vi "HDR_Query.vi"(0 "System no.":i32=1 min=1 max=4 step=1, 2 "Section header":string, 5 "error in":errorcluster) -> (14 "Data recorder help string":string, 15 "Lines":string[](array[string]), 16 "Enum values":cluster{"token string":string, i32}[](array[cluster]), 19 "error out":errorcluster)   [LabVIEW 2020]
doc: "Returns help on data recording: possible parameter values for record sources and record trigger options (DRC,DRT), parameters to set and other information. If Section header contains a valid section name, Lines and Enum values return the corresponding section content.\n\nC-887, F-206, M-8X0: Only for GCS syntax version = GCS 2.0 or higher (check with CSV?.vi. If CSV?.vi is not supported, syntax version is GCS 1.0)."
panel:
  # "Get  help for data recorder."
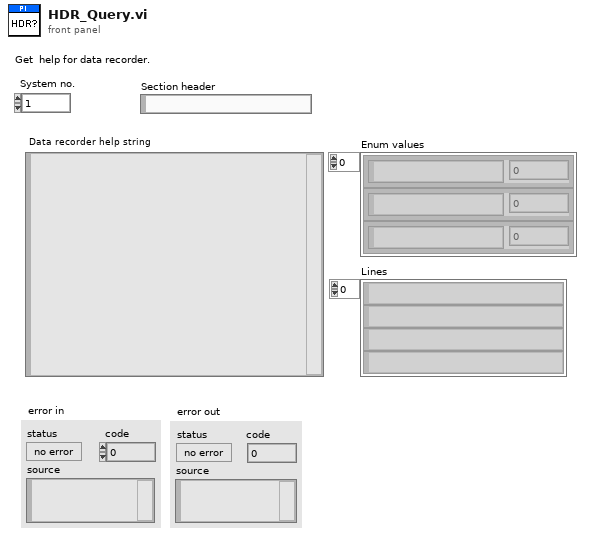
[diagram p1: front panel]
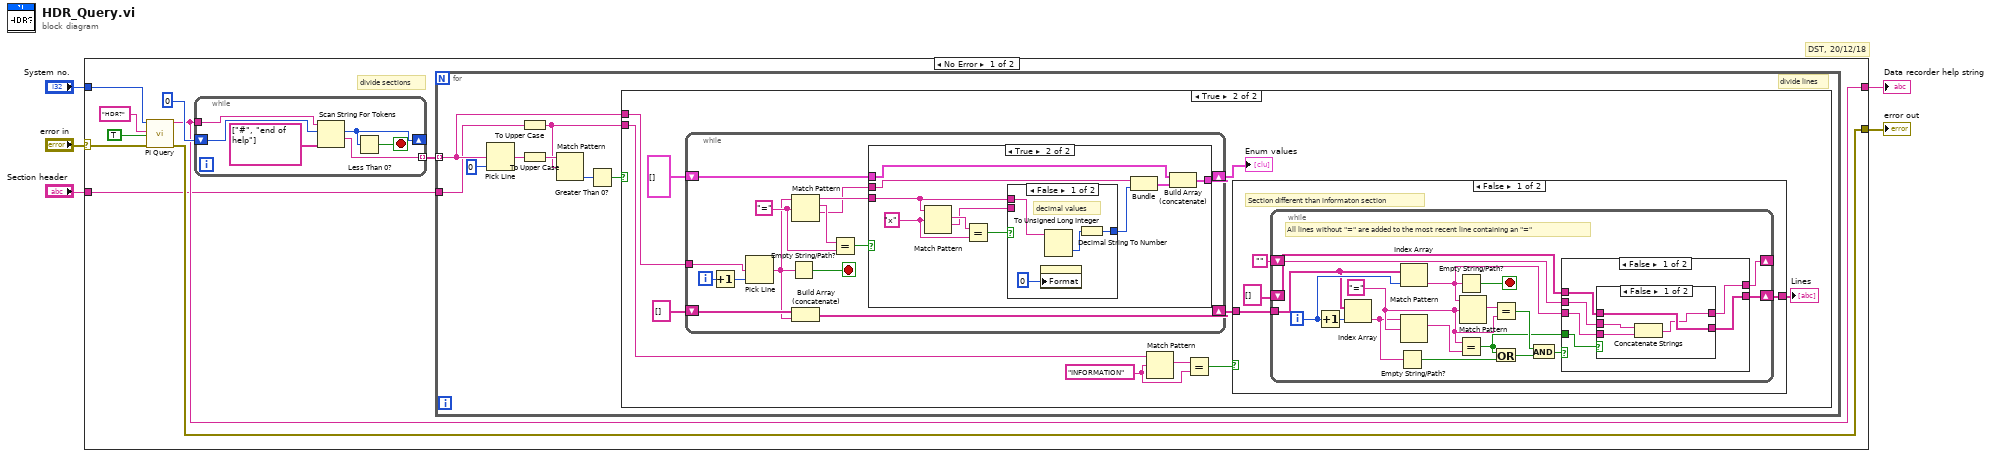
[diagram p0: block diagram]
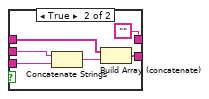
[diagram p3: hidden frame]
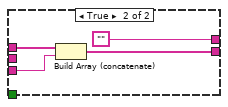
[diagram p4: hidden frame]
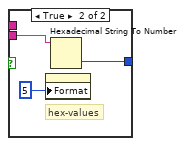
[diagram p7: hidden frame]
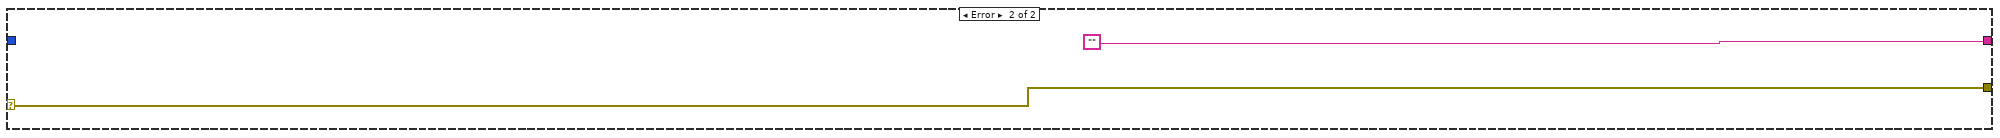
[diagram p8: hidden frame]
diagram:
  # "DST, 20/12/18"
  n1 = case shown="No Error" "error in" {
    selector: "error in" -> [w6 w115]
    tunnel: "System no." -> [w12 _]
    tunnel: [w9 "" ("String read")] -> w4
    tunnel: [w8 w115] -> w3
    tunnel: "Section header" -> [w7 _]
    frame No Error {
      # "divide sections"
      n2 = call "PI Query.vi"("System no."=w12, "String to send"="HDR?" ("String to Send"), "Attach termination char.?"=TRUE ("Attach Linefeed?"), "error in"=w6) -> ("String read"=w9:string, "error out"=w8:errorcluster)  [unwired: 3 in, 11 out]
      n3 = while {
        shift-right: [w111] -> _
        shift-left: 0 ("offset past token") -> [w113]
        tunnel: [w109] -> w10 mode=indexing
        tunnel: w9 -> [w110]
        stop <- w112 stop-if-true
        n4 = Scan String For Tokens(6:string[] ["#", "end of help"] ("delimiters (\\s,\\t,\\r,\\n)"), 8:w113, 9:w110) -> (1:w109:string, 2:w111:i32)  [unwired: 5 out]
        n5 = Less Than 0?(x=w111) -> (x < 0?=w112:bool)
      }
      n6 = for {
        tunnel: w10 -> [w21] mode=indexing
        tunnel: w7 -> [w15]
        # "divide lines"
        n7 = Pick Line(multi-line string=w21, line index=0) -> (output string=w17:string)  [unwired: 1 out]
        n8 = To Upper Case(1:w15) -> (0:w16:string)
        n9 = To Upper Case(1:w17) -> (0:w18:string)
        n10 = Match Pattern(string=w18, regular expression=w16) -> (offset past match=w19:i32)  [unwired: 4 out]
        n11 = Greater Than 0?(x=w19) -> (x > 0?=w20:bool)
        n12 = case shown="True" w20 {
          tunnel: w21 -> [_ w32]
          tunnel: w16 -> [_ w26]
          frame False {
          }
          frame True {
            w24 = "INFORMATION" ("regular expression")
            n13 = while {
              tunnel: w32 -> [w89]
              shift-right: [w80] -> w29
              shift-left: cluster{"output string":string, u16}[] [] ("array") -> [w81]
              shift-right: [w78] -> w28
              shift-left: string[] [] ("Lines") -> [w79]
              i -> [w87]
              stop <- w77 stop-if-true
              w84 = "=" ("regular expression")
              n14 = Increment(x=w87) -> (x+1=w88:i32)
              n15 = Pick Line(multi-line string=w89, line index=w88) -> (output string=w76:string)  [unwired: 1 out]
              n16 = Empty String/Path?(string/path=w76) -> (empty?=w77:bool)
              n17 = Match Pattern(string=w76, regular expression=w84) -> (before substring=w86:string, match substring=w85:string, after substring=w82:string)  [unwired: 2 out]
              n18 = Build Array (concatenate)(w79, w76) -> (w78:string[])
              n19 = Equal?(x=w85, y=w84) -> (x = y?=w83:bool)
              n20 = case shown="True" w83 {
                tunnel: w86 -> [_ w95]
                tunnel: w82 -> [_ w99]
                tunnel: w81 -> [w90 w98]
                tunnel: [w90 w96] -> w80
                frame False {
                  # "no \"=\" in the HLP answer string line\n--> line is additional info and will be ignored"
                }
                frame True {
                  w93 = "x" ("regular expression")
                  n21 = Match Pattern(string=w95, regular expression=w93) -> (match substring=w94:string, after substring=w91:string)  [unwired: 3 out]
                  n22 = Equal?(x=w94, y=w93) -> (x = y?=w92:bool)
                  n23 = case shown="False" w92 {
                    tunnel: [w103 w106] -> w100
                    tunnel: w95 -> [w104 _]
                    tunnel: w91 -> [_ w107]
                    frame False {
                      # "decimal values"
                      n24 = property class="DigNum (strict)"("Format"=u8 0 ("Display Format:Format")) -> ()  [unwired: 2 in, 2 out]
                      n25 = Decimal String To Number(string=w104) -> (number=w102:i32)  [unwired: 3 out]
                      n26 = To Unsigned Long Integer(number=w102) -> (unsigned 32bit integer=w103:u32)
                    }
                    frame True {
                      # "hex-values"
                      n27 = property class="DigNum (strict)"("Format"=u8 5 ("Display Format:Format")) -> ()  [unwired: 2 in, 2 out]
                      n28 = Hexadecimal String To Number(string=w107) -> (number=w106:u32)  [unwired: 3 out]
                    }
                  }
                  n29 = Bundle("output string"=w99, w100) -> (w97:cluster{"output string":string, u32})  [unwired: 1 out]
                  n30 = Build Array (concatenate)(w98, w97) -> (w96:cluster{"output string":string, u32}[])
                }
              }
            }
            "Enum values" <- w29
            n31 = Match Pattern(string=w26, regular expression=w24) -> (match substring=w25:string)  [unwired: 4 out]
            n32 = Equal?(x=w25, y=w24) -> (x = y?=w23:bool)
            n33 = case shown="False" w23 {
              tunnel: w28 -> [w36 w75]
              tunnel: [w34 w75] -> w27
              frame False {
                # "Section different than informaton section"
                n34 = while {
                  shift-right: [w47] -> w34
                  shift-left: string[] [] ("Lines") -> [w48]
                  shift-right: [w45] -> _
                  shift-left: "" -> [w44]
                  tunnel: w36 -> [w46]
                  i -> [w52]
                  stop <- w37 stop-if-true
                  w43 = "=" ("regular expression")
                  # "All lines without \"=\" are added to the most recent line containing an \"=\""
                  n35 = Increment(x=w52) -> (x+1=w53:i32)
                  n36 = Index Array(array=w46, index=w53) -> (element=w40:string)
                  n37 = Empty String/Path?(string/path=w40) -> (empty?=w39:bool)
                  n38 = Index Array(array=w46, index=w52) -> (element=w38:string)
                  n39 = Match Pattern(string=w40, regular expression=w43) -> (match substring=w51:string)  [unwired: 4 out]
                  n40 = Empty String/Path?(string/path=w38) -> (empty?=w37:bool)
                  n41 = Equal?(x=w43, y=w51) -> (x = y?=w42:bool)
                  n42 = Match Pattern(string=w38, regular expression=w43) -> (match substring=w54:string)  [unwired: 4 out]
                  n43 = Equal?(x=w54, y=w43) -> (x = y?=w50:bool)
                  n44 = Or(x=w42, y=w39) -> (x .or. y?=w41:bool)
                  n45 = And(x=w50, y=w41) -> (x .and. y?=w49:bool)
                  n46 = case shown="False" w49 {
                    tunnel: w38 -> [w60 w71]
                    tunnel: w48 -> [w56 w74]
                    tunnel: [w55 w73] -> w47
                    tunnel: [w59 ""] -> w45
                    tunnel: w44 -> [w58 _]
                    tunnel: w42 -> [w57 _]
                    frame False {
                      n47 = case shown="False" w57 {
                        tunnel: w60 -> [w62 w65]
                        tunnel: [w61 ""] -> w59
                        tunnel: w58 -> [w63 w66]
                        tunnel: w56 -> [w64 w69]
                        tunnel: [w64 w70] -> w55
                        frame False {
                          n48 = Concatenate Strings(w63, w62) -> (w61:string)
                        }
                        frame True {
                          n49 = Concatenate Strings(w66, w65) -> (w68:string)
                          n50 = Build Array (concatenate)(w69, w68) -> (w70:string[])
                        }
                      }
                    }
                    frame True {
                      n51 = Build Array (concatenate)(w74, w71) -> (w73:string[])
                    }
                  }
                }
              }
              frame True {
                # "If section contains only information and no options,\ndo not filter lines"
              }
            }
            "Lines" <- w27
          }
        }
      }
    }
    frame Error {
    }
  }
  "Data recorder help string" <- w4
  "error out" <- w3
